vi "Write json to AOParam one.vi"(8 "error in (no error)":errorcluster, 10 "JSON Data In":string, 11 "AO in":T1) -> (0 "error out":errorcluster, 3 "AO out":T1)   [LabVIEW 2019, in "Inputs.lvlib"]
uses:
  Inputs.lvlib
  Ctl/AO.ctl
  Ctl/Parameter State.ctl
  Ctl/AOParamColumns.ctl
  <vilib>/JDP Science/JSONtext/Find Multiple Items.vi
  <vilib>/JDP Science/JSONtext/String Subset.vi
  <vilib>/JDP Science/JSONtext/support/Strip Quotes and Unescape.vi
  <vilib>/JDP Science/JSONtext/support/Unescape JSON string.vi
  <vilib>/JDP Science/JSONtext/Parsing/Parse Full Path or Item Name.vi
  <vilib>/JDP Science/JSONtext/Offset/Find Item Locations by Path.vi
  <vilib>/JDP Science/JSONtext/Get Array Elements.vi
  Userlib.lvlib
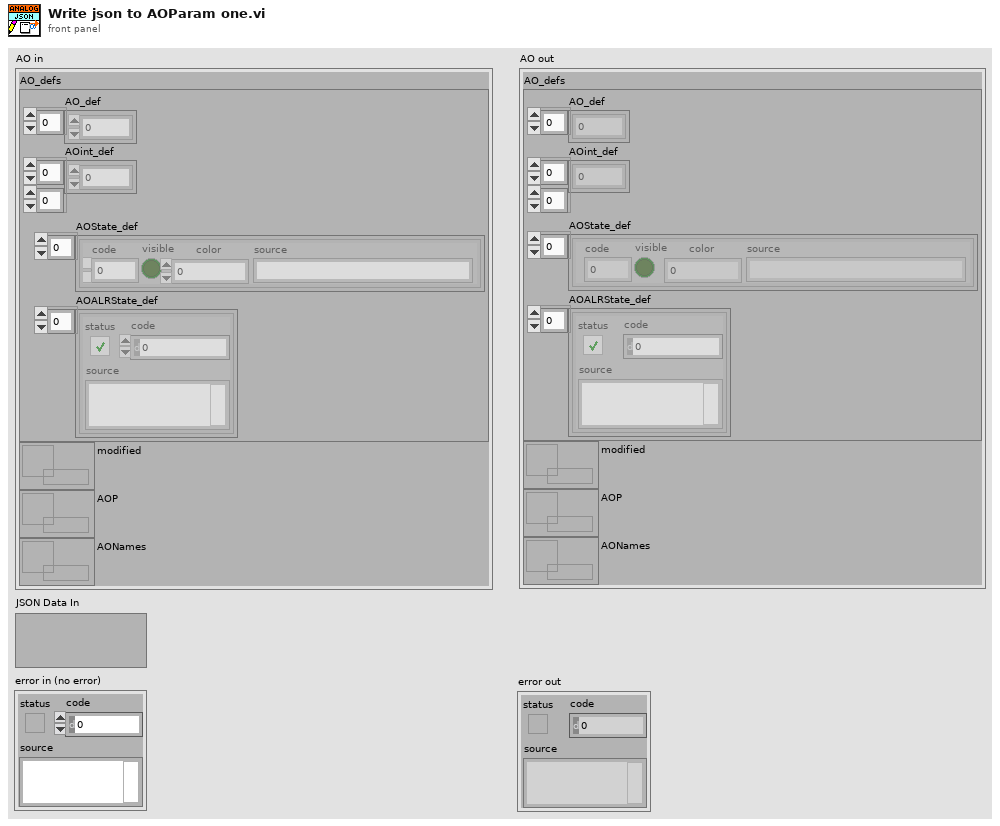
[diagram p1: front panel]
types:
  T1 = typedef "Inputs.lvlib/AO.ctl" = cluster{"AO_defs":cluster{"AO_def":dbl[], "AOint_def":u16[][], "AOState_def":T2[], "AOALRState_def":errorcluster[]}, "modified":refnum<data-value>, "AOP":refnum<data-value>, "AONames":refnum<data-value>}
  T2 = typedef "Inputs.lvlib/Parameter State.ctl" = cluster{"code":i32, "visible":bool, "color":u32, "source":string}
  T3 = typedef "Inputs.lvlib/AOParamColumns.ctl" = enum16{"instrument_gain", "instrument_offset", "instrument_range_min", "instrument_range_max", "output_pv_min", "output_pv_max", "output_register_min", "output_register_max", "module_fcode_full", "control_channel_num", "fcode", "fcodef", "fcode_full", "fname", "instrument_units"}
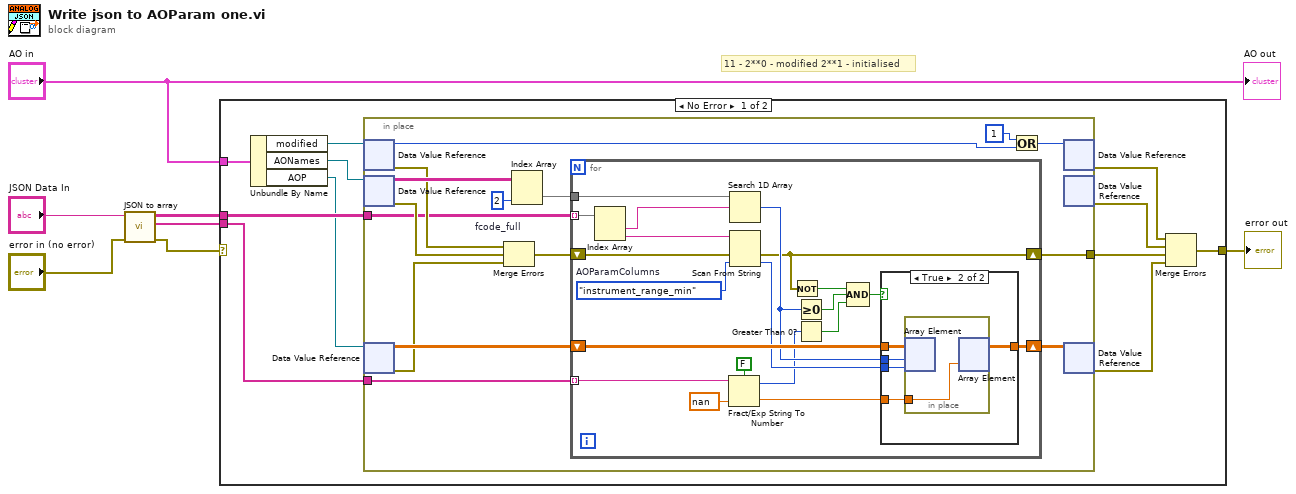
[diagram p0: block diagram]
diagram:
  # "11 - 2**0 - modified 2**1 - initialised"
  n1 = call "JSON to array.vi"("error in (no error)"="error in (no error)", "JSON Data In"="JSON Data In") -> ("error out"=w4:errorcluster, "values"=w1:string[], "names"=w2:string[][])  [unwired: 7 in]
  n2 = case shown="No Error" w4 {
    selector: w4 -> [_ w61]
    tunnel: [w17 w61] -> w7
    tunnel: "AO in" -> [w18 _]
    tunnel: w1 -> [w13 _]
    tunnel: w2 -> [w14 _]
    frame No Error {
      n3 = Unbundle By Name(w18) -> ("modified"=w16:refnum<data-value>, "AONames"=w15:refnum<data-value>, "AOP"=w12:refnum<data-value>)
      n4 = in-place {
        in-place-border: w13 -> [w26]
        in-place-border: [w27] -> w9
        in-place-border: w14 -> [w20]
        w19 = 2  # fcode_full
        n5 = in-place-dvr #1(w16) -> (w24:u8, w22:errorcluster)
        n6 = in-place-dvr #2(w15) -> (w31:string[][], w29:errorcluster)
        n7 = in-place-dvr #3(w12) -> (w33:dbl[][], w28:errorcluster)
        n8 = Merge Errors(w22, w29, w28) -> (w21:errorcluster)
        n9 = Index Array(array=w31, index (col)=w19) -> (element=w30:string[])  [unwired: 1 in]
        n10 = for {
          tunnel: w30 -> [w51]
          tunnel: w26 -> [w49] mode=indexing
          shift-right: [w35] -> w27
          shift-left: w21 -> [w46]
          shift-right: [w52] -> w32
          shift-left: w33 -> [w53]
          tunnel: w20 -> [w45] mode=indexing
          w34 = AOParamColumns."instrument_range_min"  # AOParamColumns
          n11 = Index Array(array=w45) -> (element #1=w44:string, element #2=w43:string)  [unwired: 2 in]
          n12 = Fract/Exp String To Number(use system decimal point (T)=FALSE, string=w49, default (0 dbl)=nan ("default (0 DBL)")) -> (offset past number=w40:i32, number=w48:dbl)  [unwired: 1 in]
          n13 = Search 1D Array(1D array=w51, element=w44) -> (index of element=w41:i32)  [unwired: 1 in]
          n14 = Scan From String(input string=w43, error in=w46, default 1=w34) -> (error out=w35:errorcluster, output 1=w50:T3)  [unwired: 2 in, 2 out]
          n15 = Not(x=w35) -> (.not. x?=w39:bool)
          n16 = Greater Or Equal To 0?(x=w41) -> (x >= 0?=w38:bool)
          n17 = Greater Than 0?(x=w40) -> (x > 0?=w37:bool)
          n18 = Compound Arithmetic op=AND(w39, w38, w37) -> (w36:bool)
          n19 = case shown="True" w36 {
            tunnel: w53 -> [w54 w59]
            tunnel: [w54 w58] -> w52
            tunnel: w50 -> [_ w57]
            tunnel: w48 -> [_ w56]
            tunnel: w41 -> [_ w55]
            frame False {
            }
            frame True {
              n20 = in-place {
                in-place-border: w56 -> [w60]
                n21 = in-place-array #4(w59, w55, w57) -> ()  [unwired: 1 out]
                n22 = in-place-array #4(w60) -> (w58:dbl[][])  [unwired: 2 out]
              }
            }
          }
        }
        n23 = Or(x=u8 1 ("data value"), y=w24) -> (x .or. y?=w23:u8)
        n24 = in-place-dvr #1(w23) -> (w11:errorcluster)  [unwired: 1 out]
        n25 = in-place-dvr #2() -> (w10:errorcluster)  [unwired: 1 in, 1 out]
        n26 = in-place-dvr #3(w32) -> (w8:errorcluster)  [unwired: 1 out]
      }
      n27 = Merge Errors(w11, w10, w9, w8) -> (w17:errorcluster)
    }
    frame Error {
    }
  }
  "error out" <- w7
  "AO out" <- "AO in"
